vi "Multi-Function-Synch AI-AO.vi"() -> ()   [LabVIEW 2015]
doc: "I. Description:\nThis example demonstrates how to continuously acquire and generate data at the same time, synchronized with one another.\n\nII. Instructions for Running:\n1. Select the physical channel to correspond to where your signal is input on the DAQ device. Also, select the corresponding channel for where your signal is being generated.\n2. Enter the minimum and maximum voltage ranges.\nNote: For better accuracy try to match the input range to the expected voltage level of the measured signal.\n3. Set the sample rate of the acquisition.\nNote: The rate should be at least twice as fast as the maximum frequency component of the signal being acquired. \n6. Select the Rate for the generation\n7. Select what type of signal to generate and the amplitude.\nNote: This example requires two DMA channels to run. If your hardware does not support two DMA channels, you need to set the Data Transfer Mechanism property for the Analog Output Task to use \"Interrupts\". The Data Transfer Mechanism property is located in the DAQmx Channel Property hierarchy at:\n\nDAQmx Channel Property Node>>Analog Output>>General Properties>>Advanced>>Data Transfer and Memory>>Data Transfer Mechanism\n\nRefer to your device documentation to determine how many DMA channels are supported for your hardware.\n\nIII. Block Diagram Steps:\n1. Create an analog input voltage channel. Also, create an analog output voltage channel.\n2. Set the rate for the sample clock. Additionally, define the sample mode to be continuous. Also, set the sample clock rate for the signal generation.\n2a. Call the Get Terminal Name with Device Prefix VI. This will take a Task and a terminal and create a properly formatted device + terminal name to use as the source of the Trigger.\n3. Define the parameters for a Digital Edge Start Trigger. Set the Analog output to trigger off the AI Start Trigger. This is an internal trigger signal.\n4. Use the Basic Function Generator VI to create the signal to be generated.\n5. Call the Start VI to arm the two functions. Make sure the analog output is armed before the analog input. This will ensure both will start at the same time.\n6. Read the waveform data in a loop until the user hits the stop button or an error occurs. The Is Task Done? VI is used to check for errors in the Analog Output Task.\n7. Call the Clear VI to Clear the Task\n8. Use the popup dialog box to display an error if any.\n\nIV. I/O Connections Overview:\nMake sure your signal input/output terminals match the Physical Channel I/O controls."
uses:
  <vilib>/DAQmx/configure/timing.llb/DAQmx Timing (Sample Clock).vi
  <vilib>/DAQmx/configure/trigger.llb/DAQmx Start Trigger (Digital Edge).vi
  <vilib>/DAQmx/write.llb/DAQmx Write (Analog Wfm 1Chan NSamp).vi
  <vilib>/DAQmx/create/channels.llb/DAQmx Create Channel (AO-Voltage-Basic).vi
  <vilib>/DAQmx/create/channels.llb/DAQmx Create Channel (AI-Voltage-Basic).vi
  <vilib>/DAQmx/read.llb/DAQmx Read (Analog Wfm 1Chan NSamp).vi
  <vilib>/Utility/error.llb/DialogType.ctl
  <resource>/objmgr/daqmx.rc
  <vilib>/measure/NI_MABase.lvlib
panel:
  in  "Ventetid(s)":u32
  out "Actual Update Generation Rate":dbl=5000.0 format="%0.2f"
  out "Actual Input Rate":dbl=10000.0 format="%0.2f"
  in  "rate":dbl=5000.0 caption="Update Generation Rate" format="%0.2f"
  in  "Samples to Read":i32=1000
  in  "minimum value":dbl=-10.0 caption="Output Minimum Value" format="%0.2f"
  in  "maximum value":dbl=10.0 caption="Output Maximum Value" format="%0.2f"
  in  "physical channels":tag="Dev1/ao0" caption="Output Physical Channels"
  in  "Maximum Value":dbl=10.0 caption="Input Maximum Value" format="%0.2f"
  in  "Minimum Value":dbl=-10.0 caption="Input Minimum Value" format="%0.2f"
  in  "Physical Channel":tag="Dev1/ai0" caption="Input Physical Channel"
  in  "Rate":dbl=10000.0 caption="Input Rate" format="%0.2f"
  out "Measurement":waveform(dbl)(graph)={"t0"=timestamp(3130175569.9063873 s since 1904-01-01), "dt"=9.999999999999999e-05, "Y"=[], "attributes"=variant("NI_ChannelName"=variant(string "Dev1/ai1"), "NI_UnitDescription"=variant(string "Volts"))}
  # "For instructions, select Help>>Show Context Help"
  # "Channel Parameters"
  # "Timing Parameters"
  # "Signal Generation"
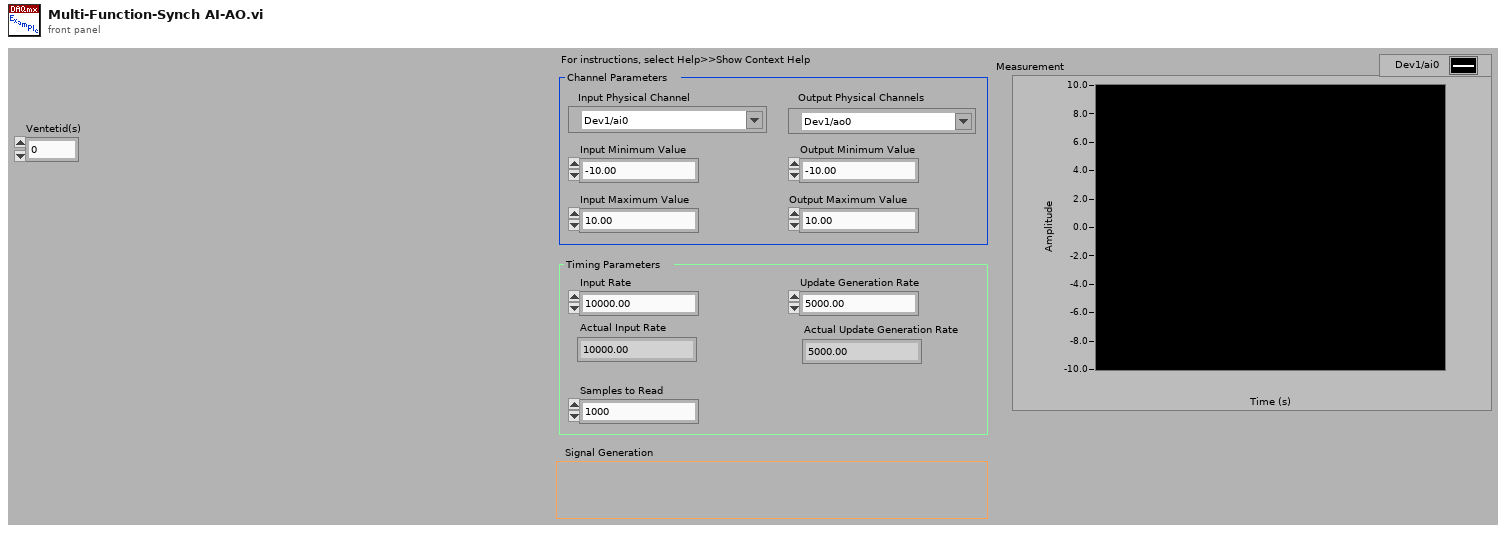
[diagram p1: front panel]
types:
  T1 = typedef "DialogType.ctl" = u16
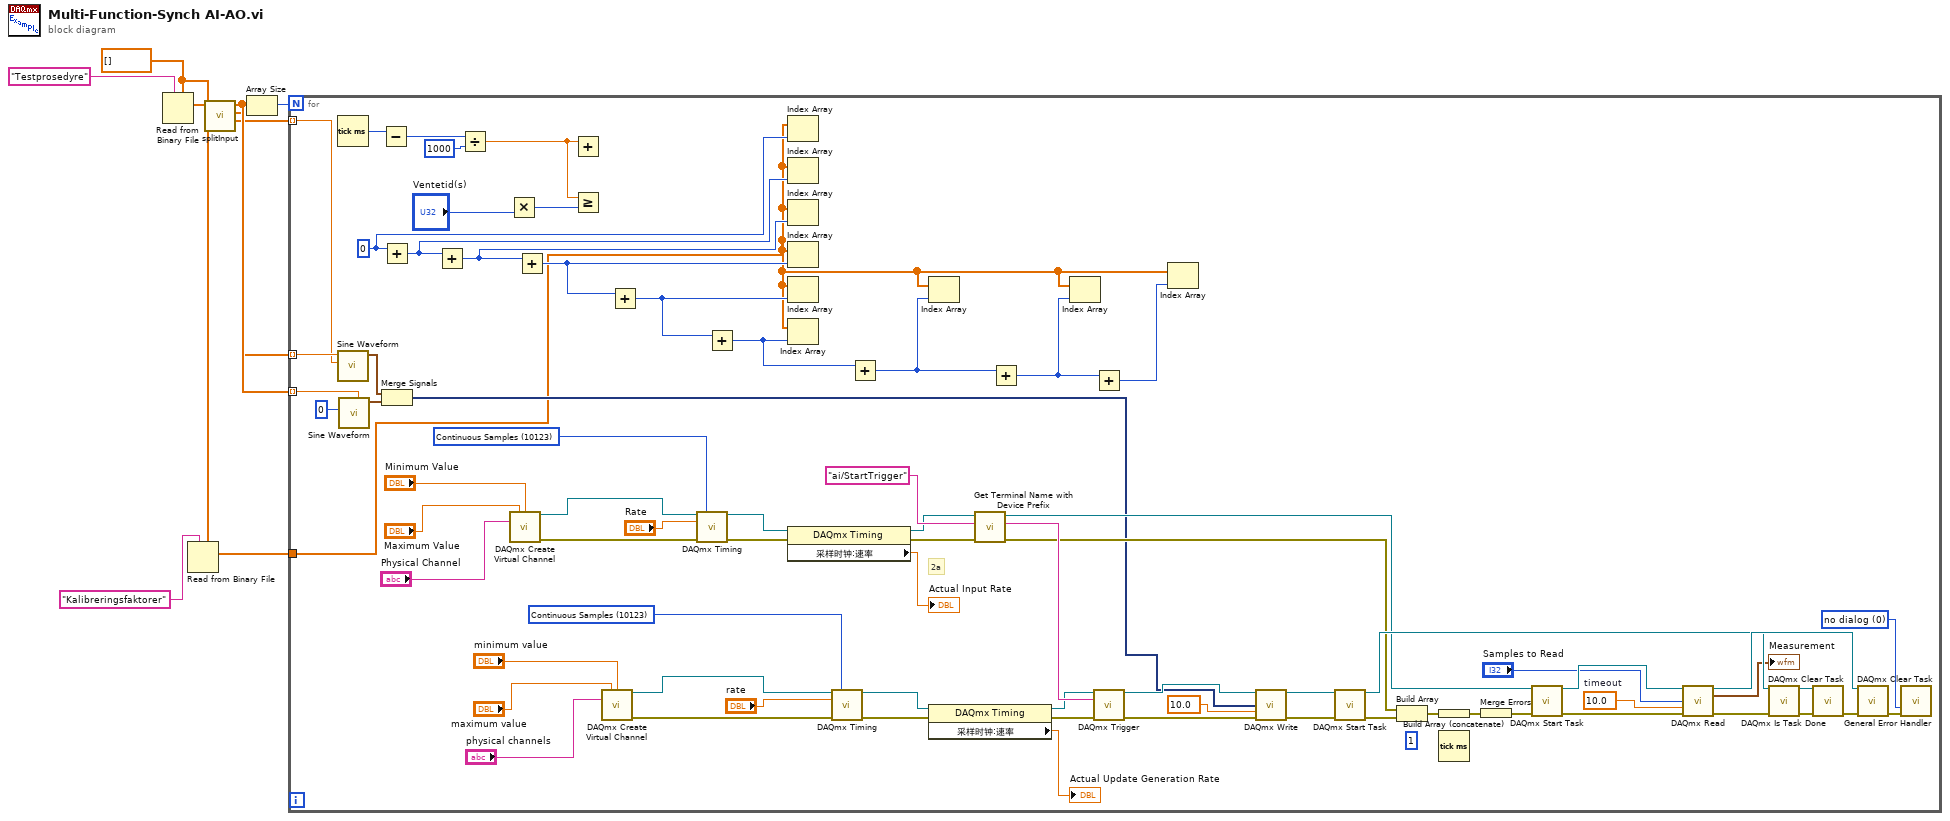
[diagram p0: block diagram]
diagram:
  w2 = dbl[] [] ("Array")
  n1 = Read from Binary File(5:w2, 7:"Testprosedyre" ("String")) -> (2:w7:dbl[])  [unwired: 4 in, 3 out]
  n2 = Read from Binary File(5:w2, 7:"Kalibreringsfaktorer") -> (2:w1:dbl[])  [unwired: 4 in, 3 out]
  n3 = call "splitInput.vi"("Array in"=w7) -> ("Amplitude"=w4:dbl[], "Frekvens"=w5:dbl[], "Temperatur"=w6:dbl[])  [unwired: 7 in, 1 out]
  n4 = Array Size(array=w6) -> (size(s)=w8:i32)
  n5 = for {
    N: w8 -> [_]
    tunnel: w6 -> [w14] mode=indexing
    tunnel: w5 -> [w13] mode=indexing
    tunnel: w4 -> [w12] mode=indexing
    tunnel: w1 -> [w10]
    (unwired) 1
    w15 = 0
    w35 = 10.0  # timeout
    w61 = T1 0 items=["no dialog", "OK message", "continue or stop message", "OK message + warnings", "continue/stop + warnings"] ("type of dialog (OK msg:1)")
    w73 = 10123 items=["Finite Samples"=10178, "Continuous Samples"=10123] ("sample mode")
    w79 = 10123 items=["Finite Samples"=10178, "Continuous Samples"=10123] ("sample mode")
    # "2a"
    n6 = Tick Count (ms)() -> (millisecond timer value=w26:u32)
    n7 = call <vilib>:"Sine Waveform.vi"("amplitude"=w12, "frequency"=w13) -> ("signal out"=w31:waveform(dbl))  [unwired: 8 in, 1 out]
    n8 = call <vilib>:"Sine Waveform.vi"("offset"=w14, "amplitude"=0) -> ("signal out"=w32:waveform(dbl))  [unwired: 8 in, 1 out]
    n9 = Subtract(x=w26) -> (x-y=w27:u32)  [unwired: 1 in]
    n10 = Add(x=w15) -> (x+y=w23:i32)  [unwired: 1 in]
    n11 = Merge Signals(w31, w32) -> (w11:dynamicdata)
    n12 = Add(x=w23) -> (x+y=w16:i32)  [unwired: 1 in]
    n13 = Divide(x=w27, y=1000) -> (x/y=w30:dbl)
    n14 = Multiply(y="Ventetid(s)") -> (x*y=w28:u32)  [unwired: 1 in]
    n15 = call-poly <vilib>:"DAQmx Create Virtual Channel.vi"("maximum value"="Maximum Value", "minimum value"="Minimum Value", "physical channels"="Physical Channel") -> ("task out"=w77:refnum<k21>, "error out"=w78:errorcluster)  [unwired: 11 in]
    n16 = Add(x=w16) -> (x+y=w17:i32)  [unwired: 1 in]
    n17 = Add(x=w30) -> ()  [unwired: 1 in, 1 out]
    n18 = Greater Or Equal?(x=w30, y=w28) -> ()  [unwired: 1 out]
    n19 = call-poly <vilib>:"DAQmx Create Virtual Channel.vi"("maximum value"="maximum value", "minimum value"="minimum value", "physical channels"="physical channels") -> ("task out"=w72:refnum<k21>, "error out"=w71:errorcluster)  [unwired: 11 in]
    n20 = Add(x=w17) -> (x+y=w18:i32)  [unwired: 1 in]
    n21 = call-poly <vilib>:"DAQmx Timing.vi"("task/channels in"=w77, "sample mode"=w79, "rate"="Rate", "error in"=w78) -> ("task out"=w46:refnum<k21>, "error out"=w45:errorcluster)  [unwired: 10 in]
    n22 = Add(x=w18) -> (x+y=w19:i32)  [unwired: 1 in]
    n23 = Index Array(array=w10, index=w15) -> ()  [unwired: 1 out]
    n24 = Index Array(array=w10, index=w23) -> ()  [unwired: 1 out]
    n25 = Index Array(array=w10, index=w16) -> ()  [unwired: 1 out]
    n26 = Index Array(array=w10, index=w17) -> ()  [unwired: 1 out]
    n27 = Index Array(array=w10, index=w18) -> ()  [unwired: 1 out]
    n28 = Index Array(array=w10, index=w19) -> ()  [unwired: 1 out]
    n29 = property class="DAQmx Timing"(reference=w46, error in=w45) -> (reference out=w44:refnum<k21>, error out=w43:errorcluster, "采样时钟:速率"=→"Actual Input Rate":dbl)
    n30 = call-poly <vilib>:"DAQmx Timing.vi"("task/channels in"=w72, "sample mode"=w73, "rate"="rate", "error in"=w71) -> ("task out"=w56:refnum<k21>, "error out"=w55:errorcluster)  [unwired: 10 in]
    n31 = Add(x=w19) -> (x+y=w20:i32)  [unwired: 1 in]
    n32 = Index Array(array=w10, index=w20) -> ()  [unwired: 1 out]
    n33 = property class="DAQmx Timing"(reference=w56, error in=w55) -> (reference out=w57:refnum<k21>, error out=w54:errorcluster, "采样时钟:速率"=→"Actual Update Generation Rate":dbl)
    n34 = call "Get Terminal Name with Device Prefix.vi"("error in (no error)"=w43, "Local Terminal Name"="ai/StartTrigger" ("terminal"), "task/channels in"=w44) -> ("error out"=w51:errorcluster, "Terminal Name with Device Prefix"=w58:tag, "task out"=w53:refnum<k21>)  [unwired: 6 in]
    n35 = Add(x=w20) -> (x+y=w21:i32)  [unwired: 1 in]
    n36 = Index Array(array=w10, index=w21) -> ()  [unwired: 1 out]
    n37 = Add(x=w21) -> (x+y=w22:i32)  [unwired: 1 in]
    n38 = call-poly <vilib>:"DAQmx Trigger.vi"("task/channels in"=w57, "source"=w58, "error in"=w54) -> ("task out"=w63:refnum<k21>, "error out"=w64:errorcluster)  [unwired: 11 in]
    n39 = Index Array(array=w10, index=w22) -> ()  [unwired: 1 out]
    n40 = call-poly <vilib>:"DAQmx Write.vi"("task/channels in"=w63, "data"=w11, "timeout"=10.0 ("Wirite Timeout"), "error in"=w64) -> ("task out"=w66:refnum<k21>, "error out"=w65:errorcluster)  [unwired: 9 in, 1 out]
    n41 = call <vilib>:"DAQmx Start Task.vi"("task/channels in"=w66, "error in"=w65) -> ("task out"=w70:refnum<k21>, "error out"=w50:errorcluster)  [unwired: 12 in]
    n42 = Build Array(w51, w50) -> (w38:errorcluster[])
    n43 = Build Array (concatenate)(w38) -> (w37:errorcluster[])
    n44 = Tick Count (ms)() -> ()  [unwired: 1 out]
    n45 = Merge Errors(w37) -> (w49:errorcluster)
    n46 = call <vilib>:"DAQmx Start Task.vi"("task/channels in"=w53, "error in"=w49) -> ("task out"=w52:refnum<k21>, "error out"=w48:errorcluster)  [unwired: 12 in]
    n47 = call-poly <vilib>:"DAQmx Read.vi"("task/channels in"=w52, "number of samples per channel"="Samples to Read", "timeout"=w35, "error in"=w48) -> ("task out"=w80:refnum<k21>, "data"=→"Measurement":waveform(dbl), "error out"=w33:errorcluster)  [unwired: 9 in]
    n48 = call <vilib>:"DAQmx Is Task Done.vi"("task/channels in"=w70, "error in"=w33) -> ("task out"=w69:refnum<k21>, "error out"=w41:errorcluster)  [unwired: 11 in, 1 out]
    n49 = call <vilib>:"DAQmx Clear Task.vi"("task in"=w69, "error in"=w41) -> ("error out"=w40:errorcluster)  [unwired: 13 in]
    n50 = call <vilib>:"DAQmx Clear Task.vi"("task in"=w80, "error in"=w40) -> ("error out"=w39:errorcluster)  [unwired: 13 in]
    n51 = call <vilib>:"General Error Handler.vi"("type of dialog (OK msg:1)"=w61, "error in (no error)"=w39) -> ()  [unwired: 9 in, 5 out]
  }
